vi "array - 副本.vi"() -> ()   [LabVIEW 2014]
uses:
  <vilib>/vision/NI_Vision_Development_Module.lvlib
panel:
  out "Image":T1(plugin-control)
  out "Image 2":T1(plugin-control)
  in  "File Path":path
  out "Pixels Values":u8[][](array[numeric])
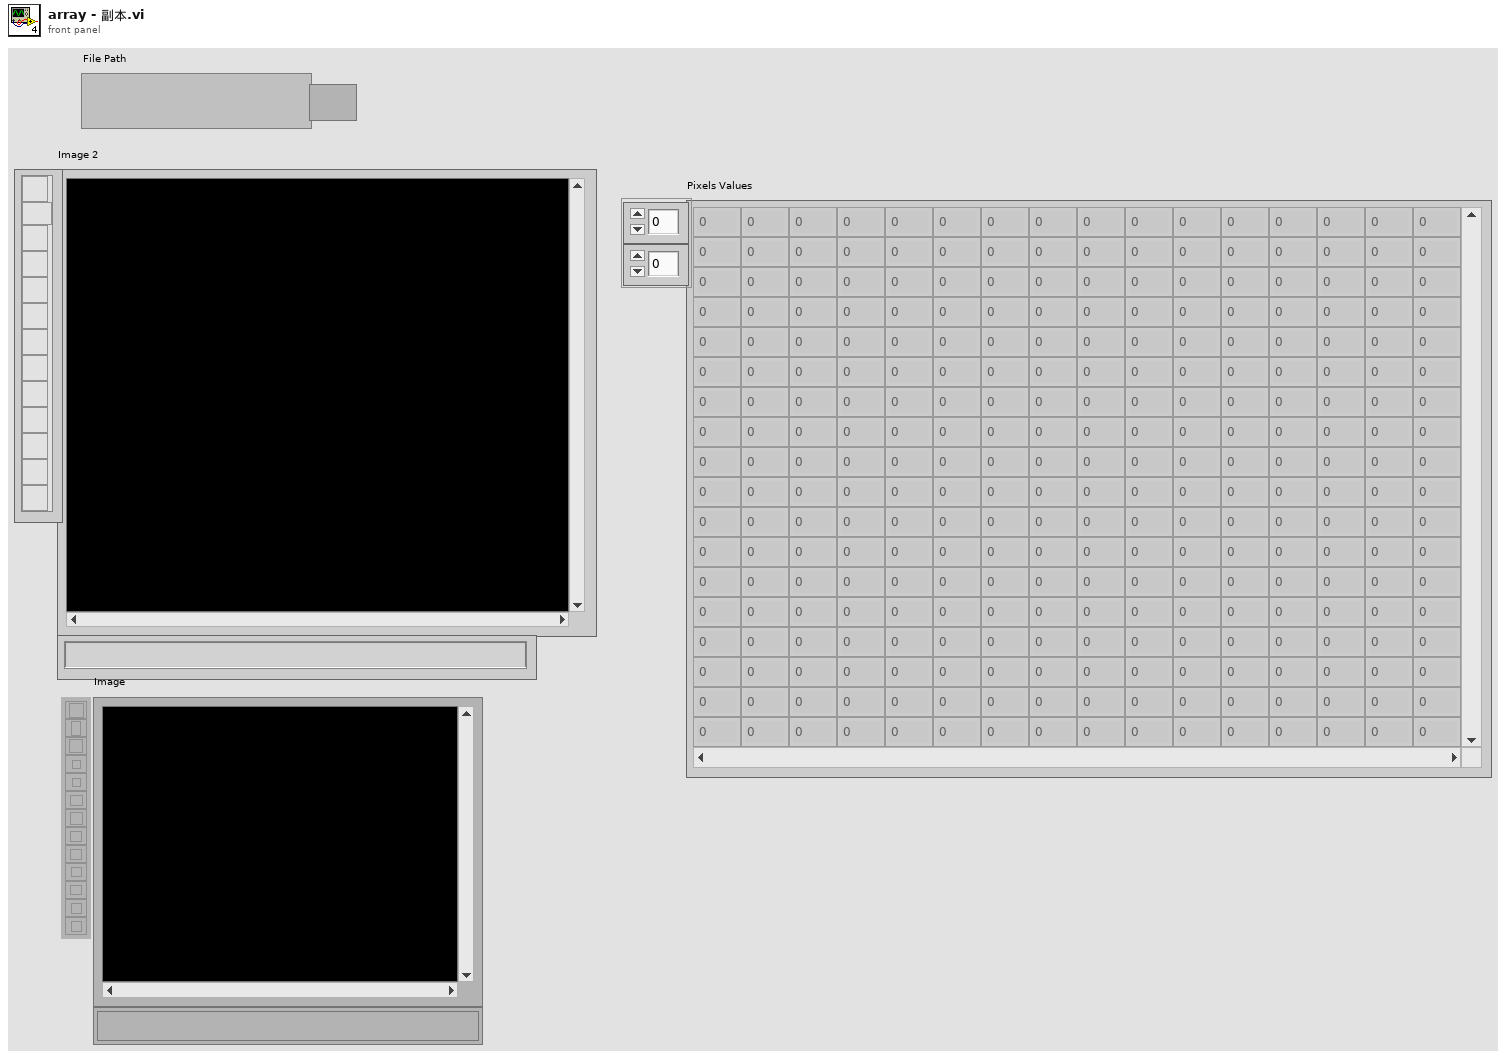
[diagram p1: front panel]
types:
  T1 = typedef "IMAQ Image.ctl" = refnum<image>
  T2 = enum32{"AutoM", "Close", "Dilate", "Erode", "Gradient", "Gradient out", "Gradient in", "Hit miss", "Open", "PClose", "POpen", "Thick", "Thin"}
  T3 = typedef "Image Type" = u32
  T4 = cluster{"Optional Rectangle[0]":i32, "Optional Rectangle[1]":i32, "Optional Rectangle[2]":i32, "Optional Rectangle[3]":i32, "Optional Rectangle[4]":i32}
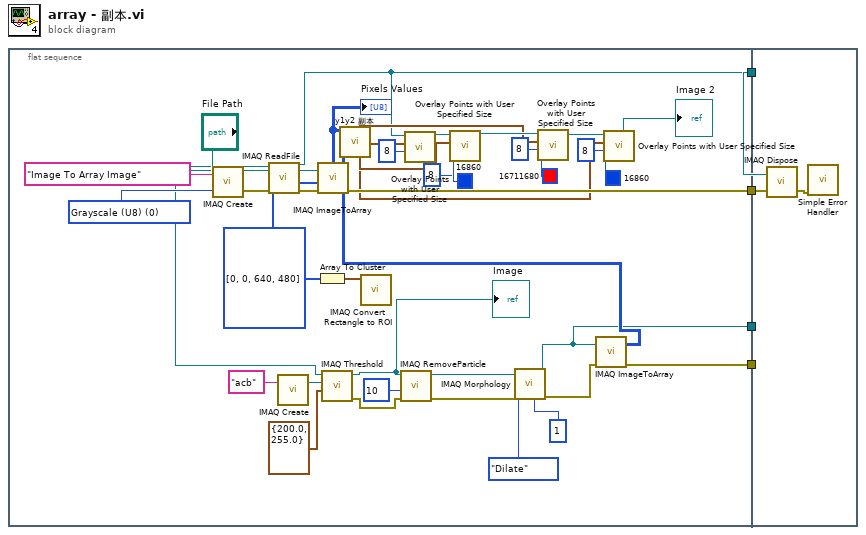
[diagram p0: block diagram]
diagram:
  n1 = flat-sequence {
    tunnel: [w21] -> w4
    tunnel: [w36] -> w3
    tunnel: [w15] -> w2
    tunnel: [w12] -> w1
    tunnel: w4 -> [w45]
    tunnel: w3 -> [w46]
    tunnel: w2 -> [_]
    tunnel: w1 -> [_]
    frame #0 {
      w35 = i32[] [0, 0, 640, 480] ("Optional Rectangle")
      w41 = T3 0 items=["Grayscale (U8)", "Grayscale (I16)", "Grayscale (SGL)", "Complex (CSG)", "RGB (U32)", "HSL (U32)", "RGB (U64)", "Grayscale (U16)"] ("Image Type")
      n2 = call "IMAQ Create"("Image Name"="Image To Array Image", "Image Type"=w41) -> ("New Image"=w42:T1, "error out"=w43:errorcluster)  [unwired: 3 in]
      n3 = call "IMAQ ReadFile"("File Path"="File Path", "error in (no error)"=w43, "Image"=w42) -> ("error out"=w40:errorcluster, "Image Out"=w21:T1)  [unwired: 4 in, 3 out]
      n4 = call "IMAQ Create"("Image Name"="acb") -> ("New Image"=w18:T1)  [unwired: 4 in, 1 out]
      n5 = Array To Cluster(array=w35) -> (cluster=w39:T4)
      n6 = call "IMAQ ImageToArray"("error in (no error)"=w40, "Optional Rectangle"=w35, "Image"=w21) -> ("error out"=w36:errorcluster, "Image Pixels (U8)"=w37:u8[][])  [unwired: 1 in, 3 out]
      "Pixels Values" <- w37
      n7 = call "IMAQ Threshold"("Range"=cluster{"Lower value":sgl, "Upper value":sgl} {"Lower value"=200.0, "Upper value"=255.0}, "Image Dst"=w18, "Image Src"=w21) -> ("error out"=w16:errorcluster, "Image Dst Out"=w5:T1)  [unwired: 7 in]
      "Image" <- w5
      n8 = call "IMAQ Convert Rectangle to ROI"("Rectangle"=w39) -> ()  [unwired: 8 in, 2 out]
      n9 = call "IMAQ RemoveParticle"("error in (no error)"=w16, "Number of Erosion"=10, "Image Src"=w5) -> ("error out"=w8:errorcluster, "Image Dst Out"=w9:T1)  [unwired: 7 in]
      n10 = call "IMAQ Morphology"("Number of iterations (1)"=1, "error in (no error)"=w8, "Operation"=T2."Dilate", "Image Src"=w9) -> ("error out"=w11:errorcluster, "Image Dst Out"=w12:T1)  [unwired: 6 in]
      n11 = call "IMAQ ImageToArray"("error in (no error)"=w11, "Image"=w12) -> ("error out"=w15:errorcluster, "Image Pixels (U8)"=w14:u8[][])  [unwired: 2 in, 3 out]
      n12 = call "y1y2 副本.vi"("二值化输入"=w14, "Image Pixels (U8)输入"=w37) -> ("out right point 2"=w22:cluster{i32, i32}[], "right"=w24:cluster{i32, i32}[], "out left point"=w23:cluster{i32, i32}[], "left"=w32:cluster{i32, i32}[])  [unwired: 3 in, 1 out]
      n13 = call "Overlay Points with User Specified Size.vi"("Point Diameter (5)"=u32 8, "Points"=w32, "Image In"=w21) -> ("Image Out"=w34:T1)  [unwired: 7 in, 1 out]
      n14 = call "Overlay Points with User Specified Size.vi"("Color"=u32 16860, "Point Diameter (5)"=u32 8, "Points"=w24, "Image In"=w34) -> ("Image Out"=w31:T1)  [unwired: 6 in, 1 out]
      n15 = call "Overlay Points with User Specified Size.vi"("Color"=u32 16711680, "Point Diameter (5)"=u32 8, "Points"=w23, "Image In"=w31) -> ("Image Out"=w30:T1)  [unwired: 6 in, 1 out]
      n16 = call "Overlay Points with User Specified Size.vi"("Color"=u32 16860, "Point Diameter (5)"=u32 8, "Points"=w22, "Image In"=w30) -> ("Image Out"=→"Image 2":T1)  [unwired: 6 in, 1 out]
    }
    frame #1 {
      n17 = call "IMAQ Dispose"("Image"=w45, "error in (no error)"=w46) -> ("error out"=w47:errorcluster)  [unwired: 4 in]
      n18 = call <vilib>:"Simple Error Handler.vi"("error in (no error)"=w47) -> ()  [unwired: 4 in, 5 out]
    }
  }
